vi "Do.vi"(8 "error in (no error)":errorcluster, 10 "Actor in":refnum<class "Actor.lvclass">, 11 "WebSocket Service Data Handler Msg":refnum<class "WebSocket Service Connection Handler Msg.lvclass">) -> (0 "error out":errorcluster, 2 "Actor out":refnum<class "Actor.lvclass">)   [LabVIEW 2016, in "WebSocket Actors.lvlib" / "WebSocket Service Connection Handler Msg.lvclass"]
doc: "(<B>Filename</B>: Actor Framework.lvlib:Message.lvclass:Do.vi)\n\nDefines what a message does when it is received by an actor. Generally, a message instructs an actor to invoke one of its methods. By default, this method does nothing. A child class must override it to define behavior. Create a child class by using the Actor Framework Message Maker dialog box."
uses:
  WebSocket Service Connection Handler Msg.lvclass
  <vilib>/ActorFramework/Actor/Actor.lvclass
  WebSocket Service/WebSocket Service.lvclass
  C:/Program Files (x86)/National Instruments/LabVIEW 2016/vi.lib/ActorFramework/Actor/Actor.lvclass
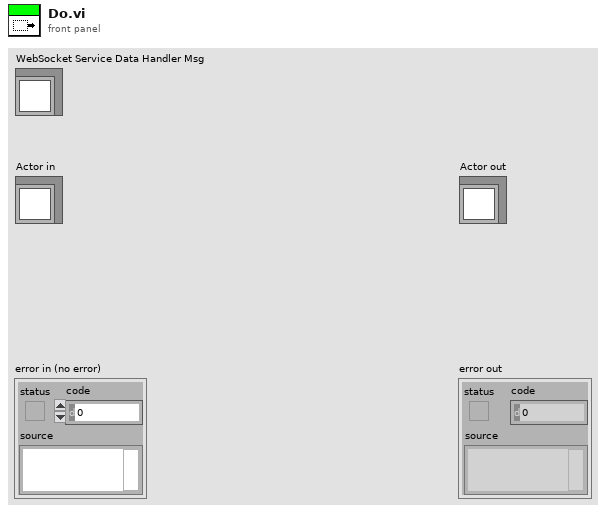
[diagram p1: front panel]
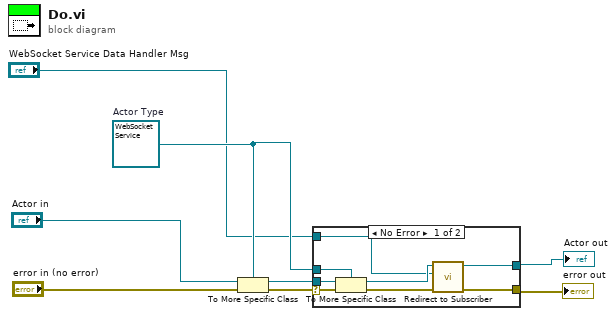
[diagram p0: block diagram]
diagram:
  w6 = refnum<class "WebSocket Service.lvclass"> refnum  # Actor Type
  n1 = To More Specific Class(target class=w6, reference="Actor in", error in="error in (no error)") -> (error out=w7:errorcluster)  [unwired: 1 out]
  n2 = case shown="No Error" w7 {
    selector: w7 -> [w15 w17]
    tunnel: [w11 w17] -> w2
    tunnel: [w10 w16] -> w4
    tunnel: "Actor in" -> [w14 w16]
    tunnel: w6 -> [w13 _]
    tunnel: "WebSocket Service Data Handler Msg" -> [w8 _]
    frame No Error {
      n3 = To More Specific Class ("Actor Cast")(target class=w13, reference=w14, error in=w15) -> (specific class reference=w9:refnum<class "WebSocket Service.lvclass">, error out=w12:errorcluster)
      n4 = call "Redirect to Subscriber.vi"("error in (no error)"=w12, "WebSocket Service Data Handler Msg"=w8, "WebSocket Service Actor in"=w9) -> ("error out"=w11:errorcluster, "WebSocket Service Actor out"=w10:refnum<class "WebSocket Service.lvclass">)  [unwired: 7 in]
    }
    frame Error {
    }
  }
  "error out" <- w2
  "Actor out" <- w4
